vi "LV FPGA Serial Write.vi"(0 "Transmit":refnum<k21>="Port8/DIO0", 1 "Write FIFO":refnum<k21>="Write FIFO", 7 "baud rate (9600)":u32=9600, 9 "data bits (8)":i32=8 min=5 max=8 step=1, 11 "parity (0:none)":enum16{"None", "Odd", "Even", "Mark", "Space"}(ring), 12 "stop bits (10: 1 bit)":u16(ring)=10 items=["1.0"=10, "1.5"=15, "2.0"=20], 13 "Invert Polarity?":bool) -> ()   [LabVIEW 2010]
uses:
  <vilib>/eio/EIOMethodNode/EIOMethodNode.xnode
  <vilib>/rvi/eio/nirviEIOMethodImplementation/nirviEIOMethodImplementation.xnode
  <vilib>/rvi/eio/common/nirviEmuClasses.ctl
  <vilib>/rvi/DataTransferAndStorage/Container/XNode/niFpgaContainer.xnode
  <vilib>/rvi/DataTransferAndStorage/Container/Common/niFpgaTransferTypeControl.ctl
  <vilib>/rvi/FIFO/Fifo_Types/niFpgaFifoControlLogicControl.ctl
  <vilib>/rvi/DataTransferAndStorage/Container/Common/niFpgaContainerMethod.ctl
  <vilib>/rvi/DataTransferAndStorage/Container/Common/niFpgaContainerMetaDataKey.ctl
  <vilib>/rvi/DataTransferAndStorage/FIFO/niFpgaPeerToPeerStreamState.ctl
  <vilib>/eio/EIONode/EIONode.xnode
  <vilib>/rvi/eio/nirviEIOImplementation/nirviEIOImplementation.xnode
  <vilib>/rvi/eio/common/nirviEmuTemplateMethod_noerrors.vi
  <vilib>/rvi/DataTransferAndStorage/Container/Common/niFpgaContainerExecOnDevCompGetState.vi
  <vilib>/rvi/FIFO/Fifo_Resource/nirvififoEmulationSetSize.vi
  <vilib>/rvi/DataTransferAndStorage/Container/Common/niFpgaContainerGetUniqueNameForEmu.vi
  <vilib>/rvi/interface/RandomDataEmulation/nirviRandomDataFPGAFIFO.vi
  <vilib>/rvi/interface/RandomDataEmulation/niFpgaRandomDataHandleErrors.vi
  <vilib>/rvi/eio/common/nirviEmuReportErrorAndStop.vi
panel:
  out "Read: Transmission Error":bool
  in  "stop":bool
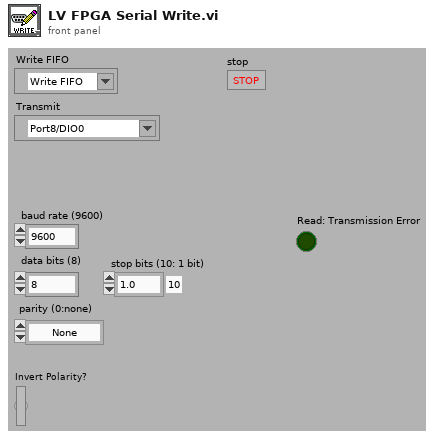
[diagram p1: front panel]
types:
  T1 = typedef "nirviEmuClasses.ctl" = enum16{"IO Read", "IO Write", "Method", "Property Read", "Property Write"}
  T2 = typedef "niFpgaFifoControlLogicControl.ctl" = enum16{"Slice Fabric", "Target Optimal", "Built-in"}
  T3 = typedef "niFpgaContainerMethod.ctl" = enum16{"<none>", "write", "read", "clear", "getNumberOfElementsToWrite", "getNumberOfElementsToRead", "enable", "disable", "flushAndDisable", "getStreamState", "readA", "readB", "dramWrite", "dramWriteWithByteEnables", "dramRequestData", "dramRetrieveData"}
  T4 = typedef "niFpgaTransferTypeControl.ctl" = enum16{"Target-Scoped", "Host to Target - DMA", "Target to Host - DMA", "Peer to Peer Reader", "Peer to Peer Writer", "Bidirectional"}
  T5 = typedef "niFpgaPeerToPeerStreamState.ctl" = enum16{"Unlinked", "Disabled", "Enabled", "Flushing"}
  T6 = typedef "niFpgaContainerMetaDataKey.ctl" = enum16{"FPGA FIFO", "FPGA Memory", "FPGA Register"}
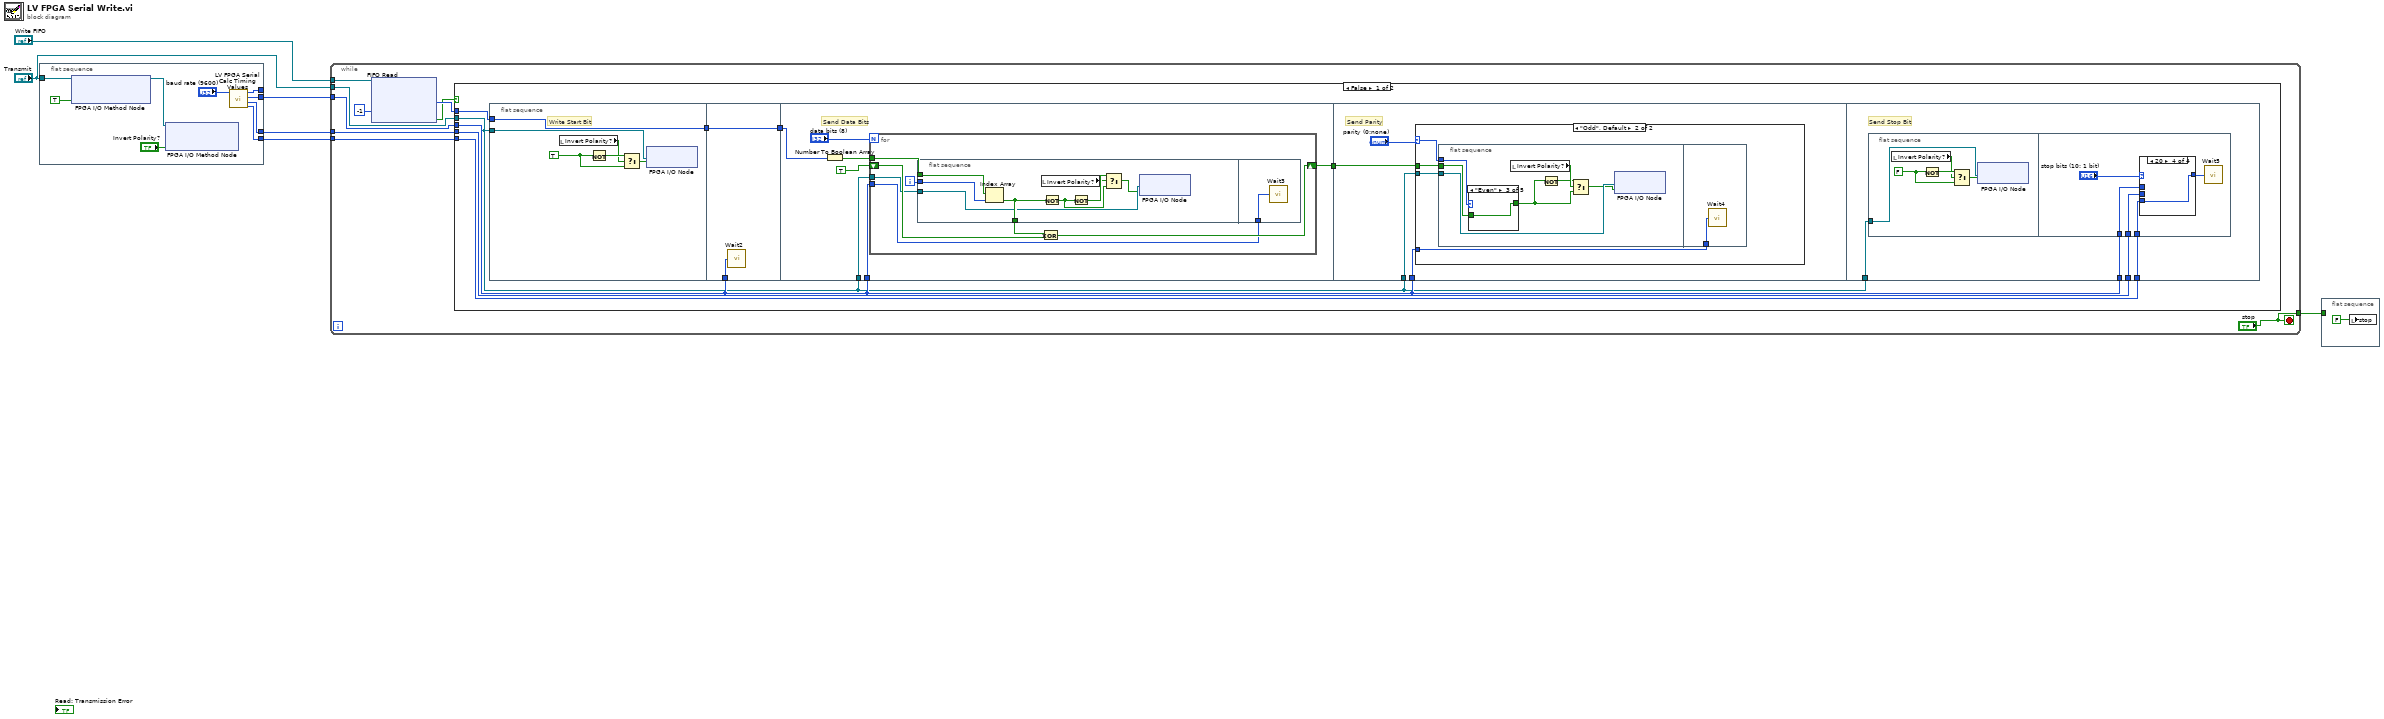
[diagram p0: block diagram]
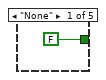
[diagram p3: hidden frame]
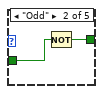
[diagram p4: hidden frame]
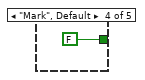
[diagram p5: hidden frame]
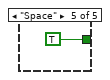
[diagram p6: hidden frame]
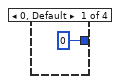
[diagram p7: hidden frame]
diagram:
  n1 = flat-sequence {
    tunnel: [w11] -> w6
    tunnel: [w14] -> _
    tunnel: [w13] -> w5
    tunnel: [w12] -> w4
    tunnel: "Transmit" -> [w9]
    frame #0 {
      n2 = xnode "FPGA I/O Method Node"("FPGA I/O In"=w9, "Enable"=TRUE ("Digital Enable")) -> ("FPGA I/O Out"=w8:refnum<k21>)
      n3 = xnode "FPGA I/O Method Node"("FPGA I/O In"=w8, "Data"="Invert Polarity?") -> ()  [unwired: 1 out]
      n4 = call "LV FPGA Serial Calc Timing Values.vi"("baud rate (1000000)"="baud rate (9600)") -> ("Two Bit"=w12:u32, "One and Half Bit"=w13:u32, "One Bit"=w11:u32, "Half Bit"=w14:u32)  [unwired: 1 in, 2 out]
    }
  }
  n5 = while {
    tunnel: w4 -> [w46]
    tunnel: w5 -> [w45]
    tunnel: w6 -> [w44]
    tunnel: "Transmit" -> [w43]
    tunnel: ["stop"] -> w2
    tunnel: "Write FIFO" -> [w39]
    stop <- "stop" stop-if-true
    n6 = xnode ("FIFO Read")("Timeout"=-1, "FIFO In"=w39) -> ("Element"=w42:u8, "Timed Out?"=w40:bool)  [unwired: 1 out]
    n7 = case shown="False" w40 {
      tunnel: w46 -> [w368 _]
      tunnel: w45 -> [w367 _]
      tunnel: w44 -> [w366 _]
      tunnel: w43 -> [w365 _]
      tunnel: w42 -> [w364 _]
      frame False {
        n8 = flat-sequence {
          tunnel: w365 -> [w377]
          tunnel: w364 -> [w372]
          tunnel: [w372] -> w371
          tunnel: w366 -> [w390]
          tunnel: [w389] -> w370
          tunnel: w371 -> [w389]
          tunnel: w366 -> [w397]
          tunnel: [w395] -> w369
          tunnel: w365 -> [w393]
          tunnel: w370 -> [w392]
          tunnel: w366 -> [w427]
          tunnel: w369 -> [w428]
          tunnel: w365 -> [w426]
          tunnel: w366 -> [w461]
          tunnel: w367 -> [w460]
          tunnel: w368 -> [w459]
          tunnel: w365 -> [w458]
          frame #0 {
            w375 = TRUE
            # "Write Start Bit"
            n9 = local read "Invert Polarity?"() -> (w374:bool)
            n10 = Not(x=w375) -> (.not. x?=w376:bool)
            n11 = Select(t=w376, s=w374, f=w375) -> (s? t:f=w373:bool)
            n12 = xnode "FPGA I/O Node"("I/O Item"=w373, "FPGA I/O In"=w377) -> ()  [unwired: 1 out]
          }
          frame #1 {
            n13 = call "Wait2"("Count(Ticks)"=w390) -> ()  [unwired: 1 out]
          }
          frame #2 {
            # "Send Data Bits"
            n14 = Number To Boolean Array(number=w392) -> (Boolean array=w394:bool[])
            n15 = for {
              N: "data bits (8)" -> [_]
              tunnel: w397 -> [w401]
              shift-right: [w404] -> w395
              shift-left: TRUE -> [w403]
              tunnel: w394 -> [w400]
              tunnel: w393 -> [w398]
              i -> [w402]
              n16 = flat-sequence {
                tunnel: w402 -> [w412]
                tunnel: w400 -> [w411]
                tunnel: [w410] -> w399
                tunnel: w398 -> [w409]
                tunnel: w401 -> [w424]
                frame #0 {
                  n17 = Index Array(array=w411, index=w412) -> (element=w410:bool)
                  n18 = local read "Invert Polarity?"() -> (w406:bool)
                  n19 = Not(x=w410) -> (.not. x?=w407:bool)
                  n20 = Not(x=w407) -> (.not. x?=w408:bool)
                  n21 = Select(t=w408, s=w406, f=w407) -> (s? t:f=w405:bool)
                  n22 = xnode "FPGA I/O Node"("I/O Item"=w405, "FPGA I/O In"=w409) -> ()  [unwired: 1 out]
                }
                frame #1 {
                  n23 = call "Wait3"("Count(Ticks)"=w424) -> ()  [unwired: 1 out]
                }
              }
              n24 = Exclusive Or(1:w403, 2:w399) -> (0:w404:bool)
            }
          }
          frame #3 {
            # "Send Parity"
            n25 = case shown="\"Odd\", Default" "parity (0:none)" {
              selector: "parity (0:none)" -> [_ w432]
              tunnel: w428 -> [_ w431]
              tunnel: w427 -> [_ w430]
              tunnel: w426 -> [_ w429]
              frame "None" {
              }
              frame "Odd", Default {
                n26 = flat-sequence {
                  tunnel: w431 -> [w438]
                  tunnel: w432 -> [w439]
                  tunnel: w429 -> [w437]
                  tunnel: w430 -> [w457]
                  frame #0 {
                    n27 = case shown="\"Even\"" w439 {
                      tunnel: w438 -> [_ w453 w454 _ _]
                      tunnel: [FALSE ("y") w452 w454 FALSE ("y") TRUE ("y")] -> w434
                      frame "None" {
                      }
                      frame "Odd" {
                        n28 = Not(x=w453) -> (.not. x?=w452:bool)
                      }
                      frame "Even" {
                      }
                      frame "Mark", Default {
                      }
                      frame "Space" {
                      }
                    }
                    n29 = local read "Invert Polarity?"() -> (w436:bool)
                    n30 = Not(x=w434) -> (.not. x?=w435:bool)
                    n31 = Select(t=w435, s=w436, f=w434) -> (s? t:f=w433:bool)
                    n32 = xnode "FPGA I/O Node"("I/O Item"=w433, "FPGA I/O In"=w437) -> ()  [unwired: 1 out]
                  }
                  frame #1 {
                    n33 = call "Wait4"("Count(Ticks)"=w457) -> ()  [unwired: 1 out]
                  }
                }
              }
            }
          }
          frame #4 {
            # "Send Stop Bit"
            n34 = flat-sequence {
              tunnel: w458 -> [w466]
              tunnel: w461 -> [w482]
              tunnel: w460 -> [w481]
              tunnel: w459 -> [w480]
              frame #0 {
                w464 = FALSE
                n35 = local read "Invert Polarity?"() -> (w463:bool)
                n36 = Not(x=w464) -> (.not. x?=w465:bool)
                n37 = Select(t=w465, s=w463, f=w464) -> (s? t:f=w462:bool)
                n38 = xnode "FPGA I/O Node"("I/O Item"=w462, "FPGA I/O In"=w466) -> ()  [unwired: 1 out]
              }
              frame #1 {
                n39 = case shown="20" "stop bits (10: 1 bit)" {
                  tunnel: w482 -> [_ w484 _ _]
                  tunnel: w481 -> [_ _ w485 _]
                  tunnel: w480 -> [_ _ _ w486]
                  tunnel: [u32 0 ("One Bit") w484 w485 w486] -> w479
                  frame 0, Default {
                  }
                  frame 10 {
                  }
                  frame 15 {
                  }
                  frame 20 {
                  }
                }
                n40 = call "Wait5"("Count(Ticks)"=w479) -> ()  [unwired: 1 out]
              }
            }
          }
        }
      }
      frame True {
      }
    }
  }
  n41 = flat-sequence {
    tunnel: w2 -> [_]
    frame #0 {
      n42 = local write "stop"(FALSE ("stop")) -> ()
    }
  }
